vi "Coerce X Output Waveform.vi"(1 "X Output Waveform":waveform(dbl)) -> (0 "Coerced X Output Waveform":waveform(dbl))   [LabVIEW 2013]
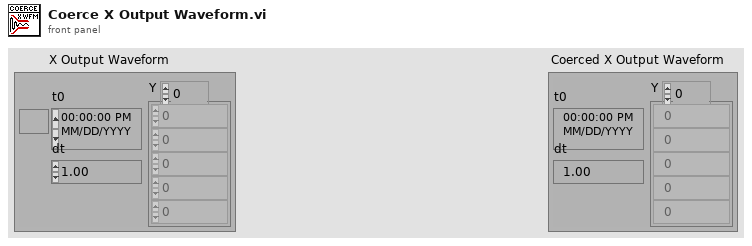
[diagram p1: front panel]
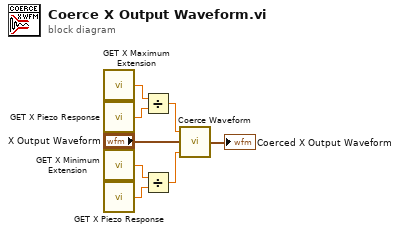
[diagram p0: block diagram]
diagram:
  n1 = call "GET X Maximum Extension.vi"() -> ("X Maximum Extension"=w5:dbl)
  n2 = call "GET X Piezo Response.vi"() -> ("X Piezo Response"=w6:dbl)
  n3 = call "GET X Minimum Extension.vi"() -> ("X Minimum Extension"=w3:dbl)
  n4 = call "GET X Piezo Response.vi"() -> ("X Piezo Response"=w4:dbl)
  n5 = Divide(x=w5, y=w6) -> (x/y=w1:dbl)
  n6 = Divide(x=w3, y=w4) -> (x/y=w2:dbl)
  n7 = call "Coerce Waveform.vi"("Lower Limit"=w2, "Output Waveform"="X Output Waveform", "Upper Limit"=w1) -> ("Coerced Output Waveform"=→"Coerced X Output Waveform":waveform(dbl))
